vi "Test Process Retains State when Stopped from Branch.vi"(8 "error in (no error)":errorcluster, 11 "Process Test In":refnum<class "Process Test.lvclass">) -> (0 "error out":errorcluster, 3 "Process Test Out":refnum<class "Process Test.lvclass">)   [LabVIEW 2020, in "Process Test.lvclass"]
uses:
  Process Test.lvclass
  Framework/Process/Process.lvclass
  Mock Error Handler/Mock Error Handler.lvclass
  <vilib>/Asteme/LUnit/Test Case.lvclass
  C:/Users/anton/Documents/GitHub/Triarc-Framework/source/Framework Test/Base Class Test/Base Test.lvclass
  C:/Program Files (x86)/National Instruments/LabVIEW 2020/vi.lib/Asteme/LUnit/Test Case.lvclass
  C:/Users/anton/Documents/GitHub/Triarc-Framework/source/Framework Test/Process Test/Process Test.lvclass
  C:/Users/anton/Documents/GitHub/Triarc-Framework/source/Framework/Process/Process.lvclass
  C:/Users/anton/Documents/GitHub/Triarc-Framework/source/Framework/Base/Base.lvclass
  C:/Users/anton/Documents/GitHub/Triarc-Framework/source/Framework/Configuration File/Configuration File.lvclass
  C:/Users/anton/Documents/GitHub/Triarc-Framework/source/Framework/Error Handler Interface/Error Handler Interface.lvclass
  C:/Users/anton/Documents/GitHub/Triarc-Framework/source/Framework Test/Mock Error Handler/Mock Error Handler.lvclass
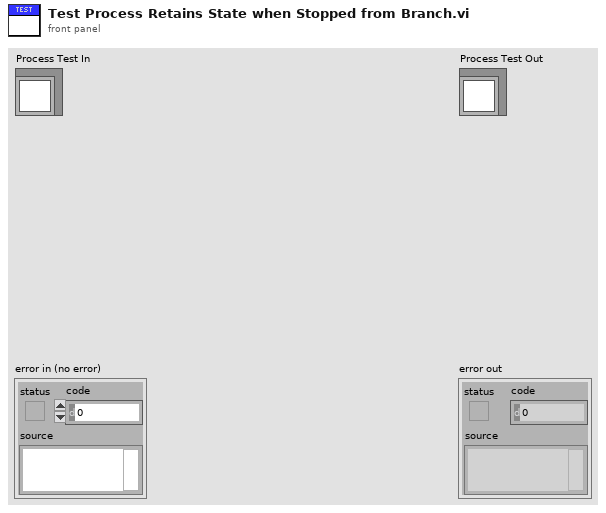
[diagram p1: front panel]
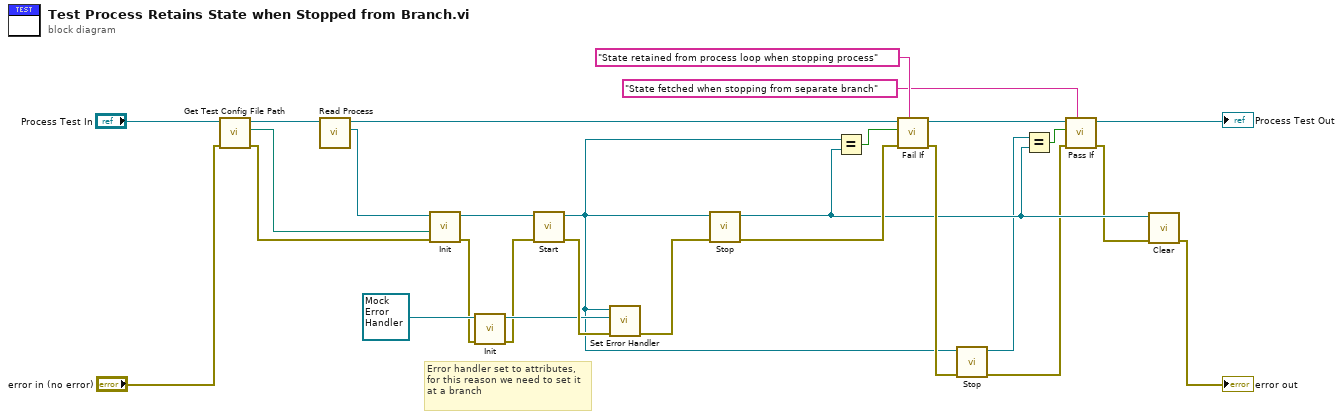
[diagram p0: block diagram]
diagram:
  # "Error handler set to attributes, for this reason we need to set it at a branch"
  n1 = call-dynamic "Get Test Config File Path.vi"("error in (no error)"="error in (no error)", "Base Class Test in"="Process Test In") -> ("error out"=w24:errorcluster, "Test config path"=w27:path, "Base Class Test out"=w28:refnum<class "Process Test.lvclass">)  [unwired: 7 in]
  n2 = call "Read Process.vi"("Process Test in"=w28) -> ("Process.lvclass"=w25:refnum<class "Process.lvclass">, "Process Test out"=w26:refnum<class "Process Test.lvclass">)  [unwired: 8 in, 1 out]
  n3 = call-dynamic "Init.vi"("error in (no error)"=w24, "Config File Path"=w27, "Process In"=w25) -> ("error out"=w13:errorcluster, "Process Out"=w17:refnum<class "Process.lvclass">)  [unwired: 7 in]
  n4 = call-dynamic "Init.vi"("error in (no error)"=w13, "Mock Error Handler In"=refnum<class "Mock Error Handler.lvclass"> refnum ("Mock Error Handler.lvclass")) -> ("error out"=w12:errorcluster, "Mock Error Handler Out"=w14:refnum<class "Mock Error Handler.lvclass">)  [unwired: 8 in]
  n5 = call "Start.vi"("error in (no error)"=w12, "Process In"=w17) -> ("error out"=w19:errorcluster, "Process Out"=w8:refnum<class "Process.lvclass">)  [unwired: 8 in]
  n6 = call "Set Error Handler.vi"("error in (no error)"=w19, "Error Handler"=w14, "Process In"=w8) -> ("error out"=w18:errorcluster)  [unwired: 7 in, 1 out]
  n7 = call "Stop.vi"("error in (no error)"=w18, "Process In"=w8) -> ("error out"=w10:errorcluster, "Process Out"=w5:refnum<class "Process.lvclass">)  [unwired: 7 in, 1 out]
  n8 = Equal?(x=w8, y=w5) -> (x = y?=w15:bool)
  n9 = call <vilib>:"Fail If.vi"("Description"="State retained from process loop when stopping process", "error in (no error)"=w10, "Fail?"=w15, "Test Case In"=w26) -> ("error out"=w9:errorcluster, "Test Case Out"=w21:refnum<class "Process Test.lvclass">)  [unwired: 6 in]
  n10 = call "Stop.vi"("error in (no error)"=w9, "Process In"=w8) -> ("error out"=w2:errorcluster, "Process Out"=w4:refnum<class "Process.lvclass">)  [unwired: 7 in, 1 out]
  n11 = Equal?(x=w4, y=w5) -> (x = y?=w3:bool)
  n12 = call <vilib>:"Pass If.vi"("Description"="State fetched when stopping from separate branch", "error in (no error)"=w2, "Pass?"=w3, "Test Case In"=w21) -> ("error out"=w1:errorcluster, "Test Case Out"=→"Process Test Out":refnum<class "Process Test.lvclass">)  [unwired: 6 in]
  n13 = call-dynamic "Clear.vi"("error in (no error)"=w1, "Process In"=w5) -> ("error out"=→"error out":errorcluster)  [unwired: 8 in, 1 out]
